vi "FCO_Read.vi"(8 "错误输入（无错误）":errorcluster caption="Error in", 11 "VISA in":refnum<visa-resource-name>) -> (0 "错误输出":errorcluster caption="Error out", 1 "Pressure(Pa)":dbl, 2 "data":string, 3 "VISA out":refnum<visa-resource-name>)   [LabVIEW 2017]
panel:
  out "Status":string
  out "Units":string
  out "Pressure":string
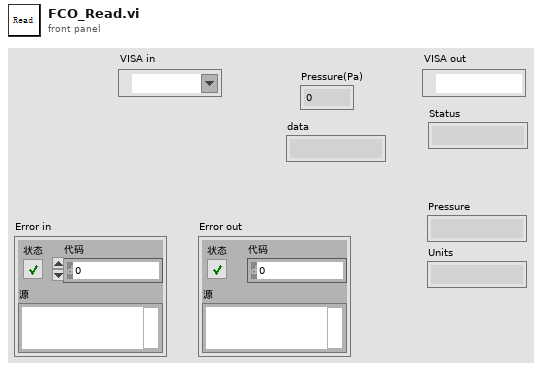
[diagram p1: front panel]
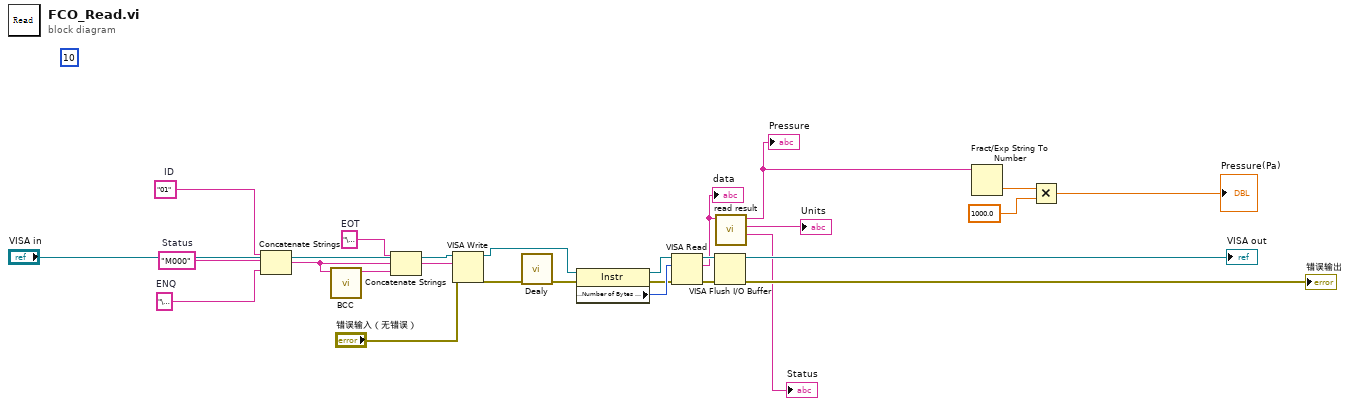
[diagram p0: block diagram]
diagram:
  w5 = "01"  # ID
  w7 = "\u0005"  # ENQ
  w10 = "M000"  # Status
  w21 = "\u0004"  # EOT
  (unwired) 10
  n1 = Concatenate Strings(w5, w10, w7) -> (w22:string)
  n2 = call "BCC.vi"("输入校验十六进制"=w22) -> ("BCC校验结果"=w23:string)  [unwired: 10 in]
  n3 = Concatenate Strings(w21, w22, w23) -> (w20:string)
  n4 = VISA Write(VISA resource name="VISA in", write buffer=w20, error in (no error)="错误输入（无错误）") -> (VISA resource name out=w12:refnum<visa-resource-name>, error out=w13:errorcluster)  [unwired: 1 out]
  n5 = call "Dealy"("error in (no error)"=w13) -> ("error out"=w18:errorcluster)  [unwired: 10 in]
  n6 = property class="Instr"(reference=w12, error in=w18) -> (reference out=w14:refnum<visa-resource-name>, error out=w15:errorcluster, "Serial Settings:Number of Bytes at Serial Port"=w16:u32)
  n7 = VISA Read(VISA resource name=w14, byte count=w16, error in (no error)=w15) -> (VISA resource name out=w19:refnum<visa-resource-name>, read buffer=w9:string, error out=w17:errorcluster)  [unwired: 1 out]
  "data" <- w9
  n8 = VISA Flush I/O Buffer(VISA resource name=w19, error in (no error)=w17) -> (VISA resource name out=→"VISA out":refnum<visa-resource-name>, error out=→"错误输出":errorcluster)  [unwired: 1 in]
  n9 = call "read result.vi"("string in"=w9) -> ("Status"=→"Status":string, "Units"=→"Units":string, "Pressure"=w4:string)  [unwired: 8 in]
  "Pressure" <- w4
  n10 = Fract/Exp String To Number(string=w4) -> (number=w3:dbl)  [unwired: 3 in, 1 out]
  n11 = Multiply(x=w3, y=1000.0) -> (x*y=→"Pressure(Pa)":dbl)
